vi "PXI-Sort Channels.vi"(9 "AO Map":T1, 11 "AI Map":T1) -> (10 "Sorted channel names":string[](array[string]), 15 "Sorted physical channels":tag[](array[tag]))   [LabVIEW 2020]
uses:
  Utility VIs/Array Dimensions (2D).vi
  <resource>/objmgr/daqmx.rc
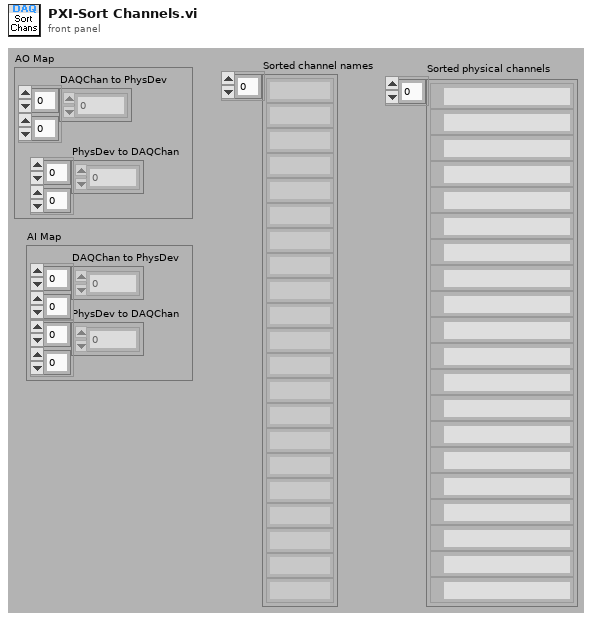
[diagram p1: front panel]
types:
  T1 = cluster{"DAQChan to PhysDev":i32[][], "PhysDev to DAQChan":i32[][]}
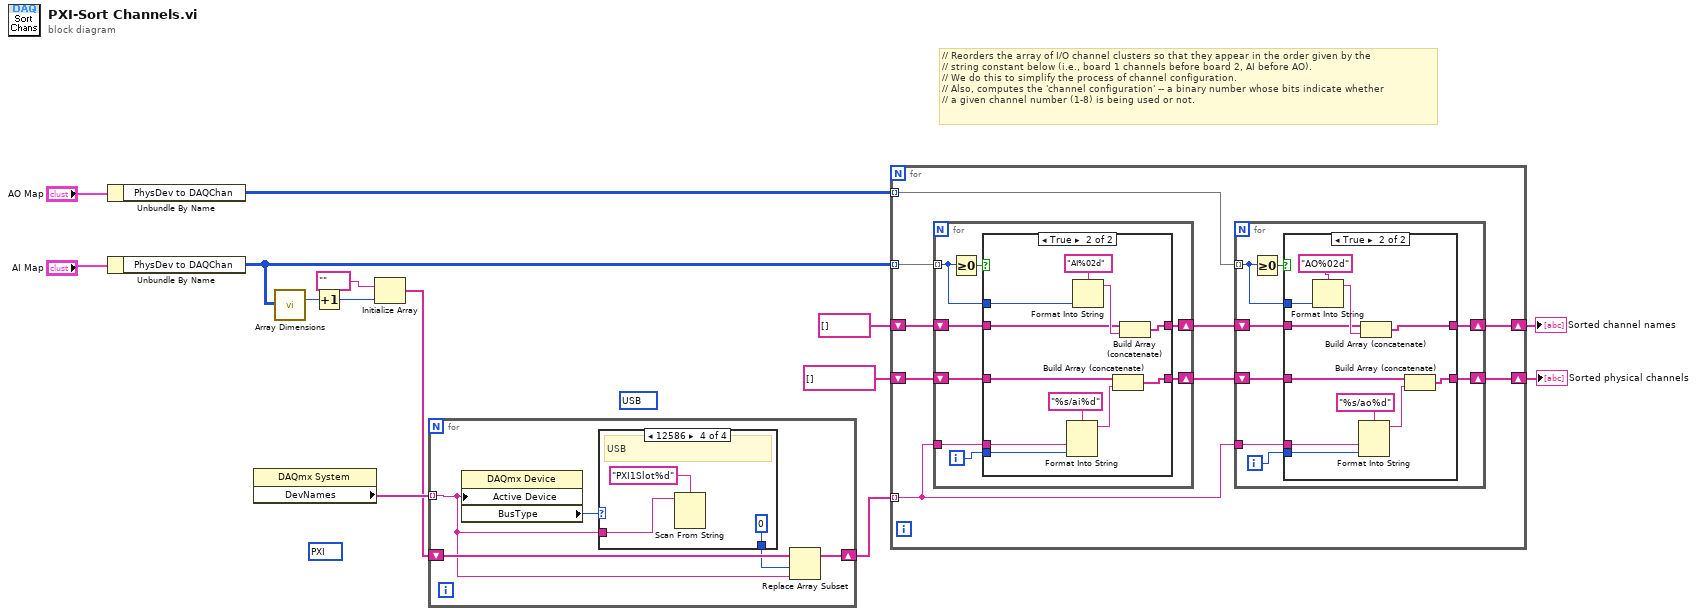
[diagram p0: block diagram]
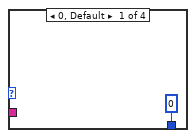
[diagram p2: hidden frame]
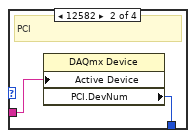
[diagram p3: hidden frame]
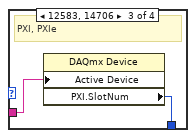
[diagram p4: hidden frame]
diagram:
  (unwired) 12586 items=["PCI"=12582, "PCIe"=13612, "PXI"=12583, "PXIe"=14706, "SCXI"=12584, "SCC"=14707, "PCCard"=12585, "USB"=12586, "CompactDAQ"=14637, "TCP/IP"=14828, "Unknown"=12588, "SwitchBlock"=15870] ("BusType")
  (unwired) 12583 items=["PCI"=12582, "PCIe"=13612, "PXI"=12583, "PXIe"=14706, "SCXI"=12584, "SCC"=14707, "PCCard"=12585, "USB"=12586, "CompactDAQ"=14637, "TCP/IP"=14828, "Unknown"=12588, "SwitchBlock"=15870] ("BusType")
  # "// Reorders the array of I/O channel clusters so that they appear in the order given by the\n// string constant below (i.e., board 1 channels before board 2, AI before AO).\n// We do this to simplify the process of channel configuration.\n// Also, computes the 'channel configuration' -- a binary number whose bits indicate whether\n// a given channel number (1-8) is being used or not."
  n1 = Unbundle By Name("AO Map") -> ("PhysDev to DAQChan"=w8:i32[][])
  n2 = Unbundle By Name("AI Map") -> ("PhysDev to DAQChan"=w2:i32[][])
  n3 = property class="DAQmx System"() -> ("DevNames"=w7:tag[])  [unwired: 2 in, 2 out]
  n4 = call-poly "Array Dimensions.vi"("2D Array"=w2) -> ("# rows"=w1:i32)  [unwired: 13 in, 1 out]
  n5 = Increment(x=w1) -> (x+1=w6:i32)
  n6 = Initialize Array(tag "" ("element"), w6) -> (w4:tag[])
  n7 = for {
    tunnel: w7 -> [w16] mode=indexing
    shift-right: [w19] -> w3
    shift-left: w4 -> [w18]
    n8 = property class="DAQmx Device"("Active Device"=w16) -> ("BusType"=w15:i32)  [unwired: 2 in, 2 out]
    n9 = case shown="12586" w15 {
      tunnel: [u32 0 ("PXI.SlotNum") w22 w24 u32 0 ("PXI.SlotNum")] -> w17
      tunnel: w16 -> [_ w21 w23 w27]
      frame 0, Default {
      }
      frame 12582 {
        # "PCI"
        n10 = property class="DAQmx Device"("Active Device"=w21) -> ("PCI.DevNum"=w22:u32)  [unwired: 2 in, 2 out]
      }
      frame 12583, 14706 {
        # "PXI, PXIe"
        n11 = property class="DAQmx Device"("Active Device"=w23) -> ("PXI.SlotNum"=w24:u32)  [unwired: 2 in, 2 out]
      }
      frame 12586 {
        # "USB"
        n12 = Scan From String(format string="PXI1Slot%d", input string=w27) -> ()  [unwired: 4 in, 3 out]
      }
    }
    n13 = Replace Array Subset(array=w18, new element=w16, index=w17) -> (w19:tag[])
  }
  n14 = for {
    tunnel: w2 -> [w36] mode=indexing
    tunnel: w8 -> [w34] mode=indexing
    shift-right: [w32] -> w11
    shift-left: string[] [] -> [w35]
    shift-right: [w29] -> w9
    shift-left: tag[] [] ("Sorted physical channels") -> [w31]
    tunnel: w3 -> [w28] mode=indexing
    n15 = for {
      tunnel: w36 -> [w64] mode=indexing
      shift-right: [w62] -> w33
      shift-left: w35 -> [w63]
      shift-right: [w60] -> w30
      shift-left: w31 -> [w61]
      tunnel: w28 -> [w59]
      i -> [w58]
      n16 = Greater Or Equal To 0?(x=w64) -> (x >= 0?=w65:bool)
      n17 = case shown="True" w65 {
        tunnel: w64 -> [_ w77]
        tunnel: w63 -> [w67 w75]
        tunnel: [w67 w74] -> w62
        tunnel: w61 -> [w66 w72]
        tunnel: [w66 w73] -> w60
        tunnel: w59 -> [_ w69]
        tunnel: w58 -> [_ w68]
        frame False {
        }
        frame True {
          n18 = Format Into String(format string="%s/ai%d", w69, w68) -> (resulting string=w71:string)  [unwired: 2 in, 1 out]
          n19 = Format Into String(format string="AI%02d", w77) -> (resulting string=w76:string)  [unwired: 2 in, 1 out]
          n20 = Build Array (concatenate)(w72, w71) -> (w73:string[])
          n21 = Build Array (concatenate)(w75, w76) -> (w74:string[])
        }
      }
    }
    n22 = for {
      tunnel: w34 -> [w43] mode=indexing
      shift-right: [w41] -> w32
      shift-left: w33 -> [w42]
      shift-right: [w39] -> w29
      shift-left: w30 -> [w40]
      tunnel: w28 -> [w38]
      i -> [w37]
      n23 = Greater Or Equal To 0?(x=w43) -> (x >= 0?=w44:bool)
      n24 = case shown="True" w44 {
        tunnel: w43 -> [_ w56]
        tunnel: w42 -> [w46 w54]
        tunnel: [w46 w53] -> w41
        tunnel: w40 -> [w45 w50]
        tunnel: [w45 w49] -> w39
        tunnel: w38 -> [_ w48]
        tunnel: w37 -> [_ w47]
        frame False {
        }
        frame True {
          n25 = Format Into String(format string="AO%02d", w56) -> (resulting string=w55:string)  [unwired: 2 in, 1 out]
          n26 = Format Into String(format string="%s/ao%d", w48, w47) -> (resulting string=w52:string)  [unwired: 2 in, 1 out]
          n27 = Build Array (concatenate)(w54, w55) -> (w53:string[])
          n28 = Build Array (concatenate)(w50, w52) -> (w49:string[])
        }
      }
    }
  }
  "Sorted channel names" <- w11
  "Sorted physical channels" <- w9
